vi "Add Director.vi"(8 "error in (no error)":errorcluster, 9 "Index":i32=-1 min=-1 step=1, 10 "Command Director":refnum<class "CommandDirector.lvclass">, 11 "InteractionProcessor in":refnum<class "InteractionProcessor.lvclass">) -> (0 "error out":errorcluster, 3 "InteractionProcessor out":refnum<class "InteractionProcessor.lvclass">)   [LabVIEW 2023, in "HAF.lvlib" / "InteractionProcessor.lvclass"]
doc: "Adds a CommandDirector into the collection for processing. The Director can be added in at a specific index; use -1 (default) to add at the end."
uses:
  InteractionProcessor.lvclass
  CommandDirector/CommandDirector.lvclass
  InteractionProcessor.lvclass/InteractionProcessor.ctl
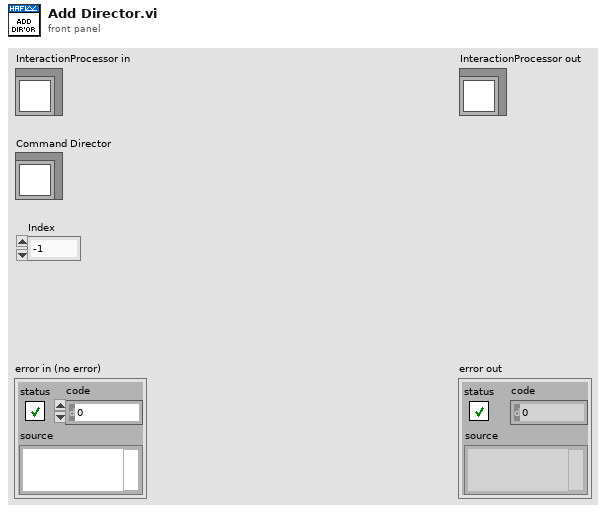
[diagram p1: front panel]
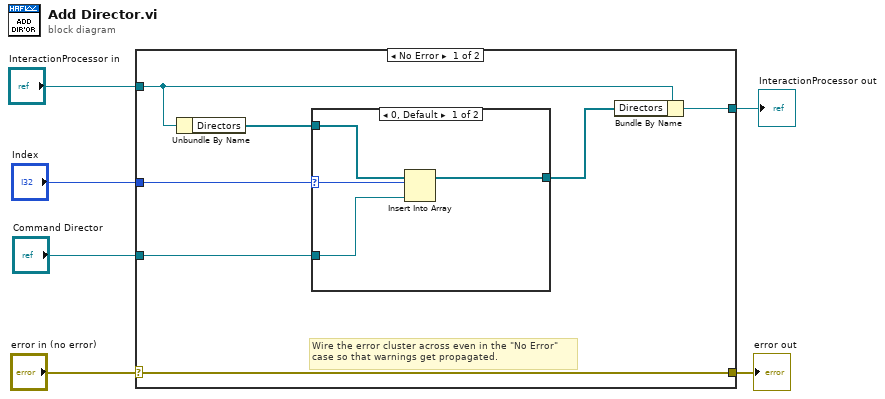
[diagram p0: block diagram]
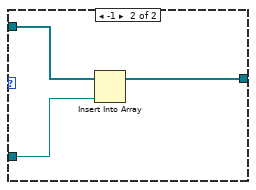
[diagram p2: hidden frame]
diagram:
  n1 = case shown="No Error" "error in (no error)" {
    selector: "error in (no error)" -> [w13 w22]
    tunnel: [w13 w22] -> w5
    tunnel: [w8 w21] -> w3
    tunnel: "InteractionProcessor in" -> [w9 w21]
    tunnel: "Index" -> [w11 _]
    tunnel: "Command Director" -> [w10 _]
    frame No Error {
      # "Wire the error cluster across even in the \"No Error\"\ncase so that warnings get propagated."
      n2 = Unbundle By Name(w9) -> ("Directors"=w12:refnum<class "CommandDirector.lvclass">[])
      n3 = case shown="0, Default" w11 {
        selector: w11 -> [w17 _]
        tunnel: w12 -> [w15 w20]
        tunnel: w10 -> [w16 w19]
        tunnel: [w14 w18] -> w7
        frame 0, Default {
          n4 = Insert Into Array(array=w15, index=w17, new element=w16) -> (w14:refnum<class "CommandDirector.lvclass">[])
        }
        frame -1 {
          n5 = Insert Into Array(array=w20, new element=w19) -> (w18:refnum<class "CommandDirector.lvclass">[])  [unwired: 1 in]
        }
      }
      n6 = Bundle By Name(cluster=w9, "Directors"=w7) -> (w8:refnum<class "InteractionProcessor.lvclass">)
    }
    frame Error {
    }
  }
  "error out" <- w5
  "InteractionProcessor out" <- w3
